vi "Add Digit.vi"(8 "error in (no error)":errorcluster, 9 "Input Array":u16[](array[numeric]), 11 "Digit":u8 max=9) -> (0 "error out":errorcluster, 1 "Output Array":u16[](array[numeric]))   [LabVIEW 2015]
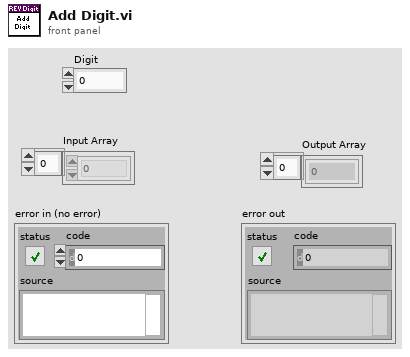
[diagram p1: front panel]
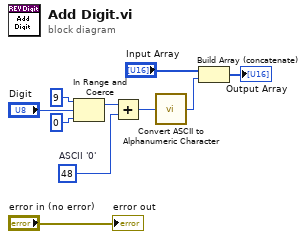
[diagram p0: block diagram]
diagram:
  w5 = u8 48  # ASCII '0'
  n1 = In Range and Coerce(upper limit=u8 9, x="Digit", lower limit=u8 0) -> (coerced(x)=w3:u8)  [unwired: 1 out]
  n2 = Add(x=w3, y=w5) -> (x+y=w6:u8)
  n3 = call "Convert ASCII to Alphanumeric Character.vi"("ASCII Value"=w6) -> ("Alphanumeric Character Value"=w7:u16)
  n4 = Build Array (concatenate)("Input Array", w7) -> (→"Output Array":u16[])
  "error out" <- "error in (no error)"
